vi "Build Header.vi"(8 "error in (no error)":errorcluster {"code" format="Error %.0f"}) -> (0 "error out":errorcluster {"code" format="Error %.0f"}, 1 "File Path Out":string, 2 "Header":string, 3 "File Ref Out":refnum<file>)   [LabVIEW 2017]
panel:
  in  "End Process":bool
  in  "Comments":string
  in  "Operator":string
  in  "Customer":string
  in  "Description*":string
  in  "Test ID*":string
  in  "SPN*":string
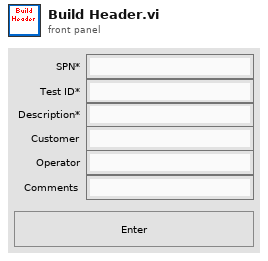
[diagram p1: front panel]
types:
  T1 = enum16{"open", "replace", "create", "open or create", "replace or create", "replace or create with confirmation"}
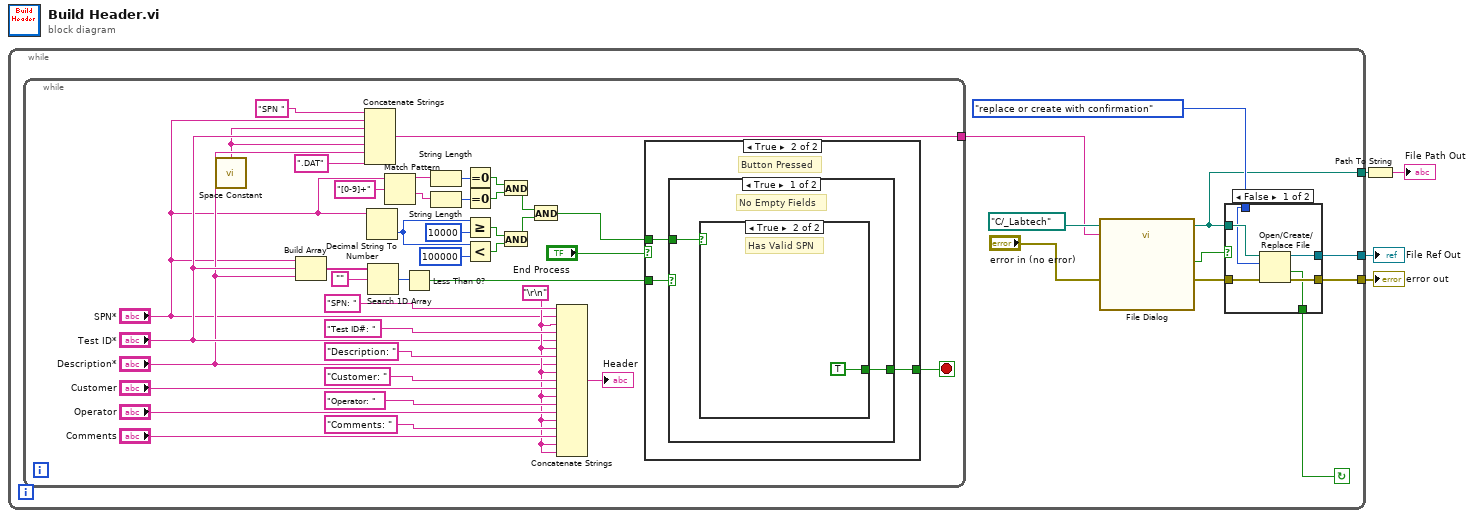
[diagram p0: block diagram]
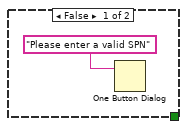
[diagram p4: hidden frame]
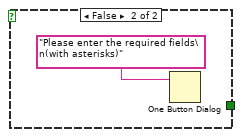
[diagram p5: hidden frame]
diagram:
  n1 = while {
    tunnel: [w9] -> w4
    tunnel: [w8] -> w3
    tunnel: [w5] -> w2
    stop <- w6 continue-if-true
    n2 = while {
      tunnel: [w40] -> w13
      stop <- w56 stop-if-true
      w46 = "\r\n"
      n3 = call <vilib>:"Space Constant.vi"() -> ("String"=w42:string)
      n4 = Build Array("SPN*", "Test ID*", "Description*") -> (w60:string[])
      n5 = Concatenate Strings("SPN ", "SPN*", w42, "Test ID*", w42, "Description*", ".DAT") -> (w40:string)
      n6 = Decimal String To Number(string="SPN*") -> (number=w35:i32)  [unwired: 2 in, 1 out]
      n7 = Search 1D Array(1D array=w60, element="") -> (index of element=w58:i32)  [unwired: 1 in]
      n8 = Match Pattern(string="SPN*", regular expression="[0-9]+") -> (before substring=w29:string, after substring=w30:string)  [unwired: 1 in, 2 out]
      n9 = Less Than 0?(x=w58) -> (x < 0?=w24:bool)
      n10 = String Length(string=w29) -> (length=w31:i32)
      n11 = String Length(string=w30) -> (length=w32:i32)
      n12 = Equal To 0?(x=w31) -> (x = 0?=w33:bool)
      n13 = Equal To 0?(x=w32) -> (x = 0?=w34:bool)
      n14 = Greater Or Equal?(x=w35, y=10000) -> (x >= y?=w37:bool)
      n15 = Less?(x=w35, y=100000) -> (x < y?=w38:bool)
      n16 = And(x=w33, y=w34) -> (x .and. y?=w36:bool)
      n17 = And(x=w37, y=w38) -> (x .and. y?=w39:bool)
      n18 = And(x=w36, y=w39) -> (x .and. y?=w23:bool)
      n19 = Concatenate Strings("SPN: ", "SPN*", w46, "Test ID#: ", "Test ID*", w46, "Description: ", "Description*", w46, "Customer: ", "Customer", w46, "Operator: ", "Operator", w46, "Comments: ", "Comments", w46, w46) -> (→"Header":string)
      n20 = case shown="True" "End Process" {
        tunnel: [_ w64] -> w56
        tunnel: w24 -> [_ w63]
        tunnel: w23 -> [_ w62]
        frame False {
        }
        frame True {
          # "Button Pressed"
          n21 = case shown="True" w63 {
            tunnel: [w65 _] -> w64
            tunnel: w62 -> [w66 _]
            frame True {
              # "No Empty Fields"
              n22 = case shown="True" w66 {
                tunnel: [_ TRUE] -> w65
                frame False {
                  n23 = One Button Dialog(message="Please enter a valid SPN") -> ()  [unwired: 1 in, 1 out]
                }
                frame True {
                  # "Has Valid SPN"
                }
              }
            }
            frame False {
              n24 = One Button Dialog(message="Please enter the required fields\n(with asterisks)") -> ()  [unwired: 1 in, 1 out]
            }
          }
        }
      }
    }
    n25 = call "File Dialog"("start path"=path "C:/_Labtech", "default name"=w13, "error in"="error in (no error)") -> ("selected path"=w5:path, "cancelled"=w7:bool, "error out"=w11:errorcluster)  [unwired: 9 in, 1 out]
    n26 = case shown="False" w7 {
      selector: w7 -> [_ w22]
      tunnel: w5 -> [w20 _]
      tunnel: w11 -> [w19 w21]
      tunnel: T1."replace or create with confirmation" ("operation (0:open)") -> [w18 _]
      tunnel: [w17 w21] -> w9
      tunnel: [w16 _] -> w8
      tunnel: [w15 w22] -> w6
      frame False {
        n27 = Open/Create/Replace File(file path (use dialog)=w20, error in=w19, operation (0:open)=w18) -> (refnum out=w16:refnum<file>, cancelled=w15:bool, error out=w17:errorcluster)  [unwired: 3 in]
      }
      frame True {
      }
    }
  }
  "error out" <- w4
  "File Ref Out" <- w3
  n28 = Path To String(path=w2) -> (string=→"File Path Out":string)
